vi "例7,1.vi"() -> ()   [LabVIEW 2017]
panel:
  out "7（X0=10.dx=2,Y）单条曲线":cluster{i32, i32, cluster{dbl[]}[]}(graph)
  out "6（X0=10.dx=2,Y）单条曲线":cluster{i32, i32, dbl[][]}(graph)
  out "5（X0=10.dx=2,Y）单条曲线":cluster{i32, i32, dbl[]}[](graph)
  out "4（X0=10.dx=2,Y）单条曲线":cluster{i32, i32, dbl[]}(graph)
  out "3（Y）单条曲线":cluster{dbl[]}[](graph)
  out "2（Y）多条曲线":dbl[][](graph)
  out "1（Y）单条曲线":dbl[](graph)
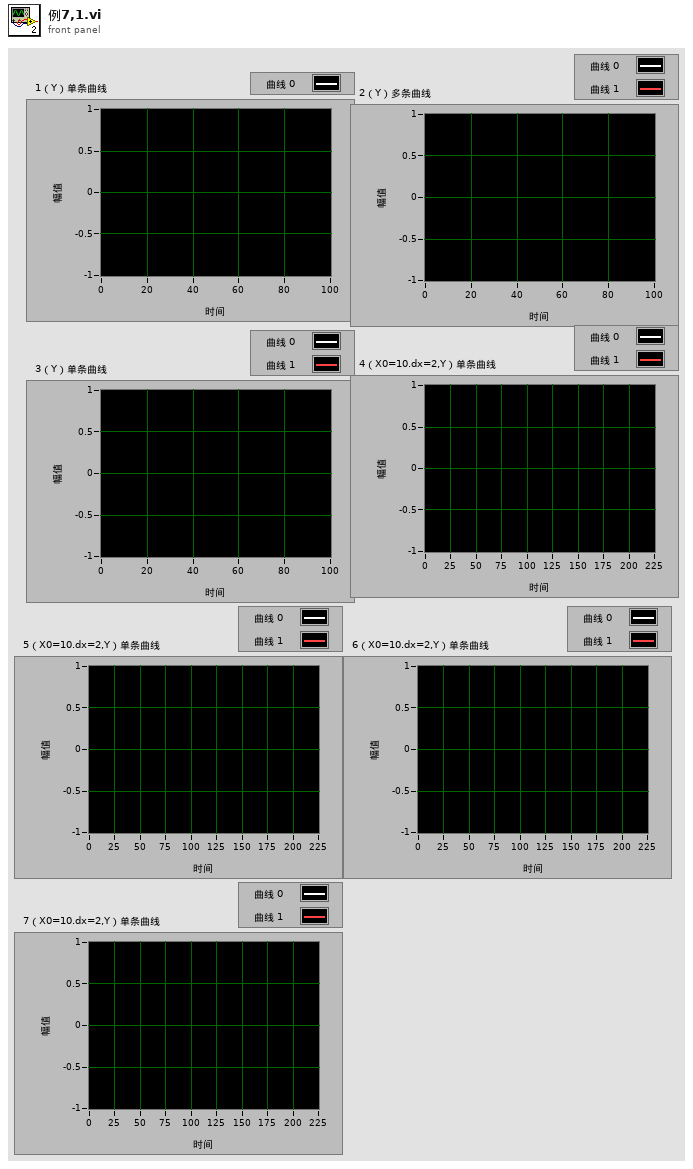
[diagram p1: front panel]
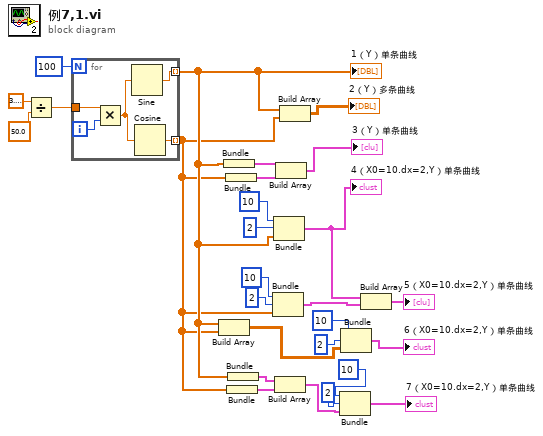
[diagram p0: block diagram]
diagram:
  n1 = Divide(x=3.141592653589793, y=50.0) -> (x/y=w25:dbl)
  n2 = for {
    N: 100 -> [_]
    tunnel: w25 -> [w31]
    tunnel: [w29] -> w19 mode=indexing
    tunnel: [w28] -> w23 mode=indexing
    i -> [w32]
    n3 = Multiply(x=w31, y=w32) -> (x*y=w30:dbl)
    n4 = Sine(x=w30) -> (sin(x)=w28:dbl)
    n5 = Cosine(x=w30) -> (cos(x)=w29:dbl)
  }
  "1（Y）单条曲线" <- w23
  n6 = Build Array(w23, w19) -> (w11:dbl[][])
  n7 = Bundle(w23) -> (w22:cluster{dbl[]})  [unwired: 1 in]
  n8 = Bundle(w19) -> (w21:cluster{dbl[]})  [unwired: 1 in]
  n9 = Bundle(w19) -> (w17:cluster{dbl[]})  [unwired: 1 in]
  n10 = Bundle(w23) -> (w18:cluster{dbl[]})  [unwired: 1 in]
  n11 = Bundle(10, 2, w19) -> (w8:cluster{i32, i32, dbl[]})  [unwired: 1 in]
  n12 = Bundle(10, 2, w23) -> (w12:cluster{i32, i32, dbl[]})  [unwired: 1 in]
  "4（X0=10.dx=2,Y）单条曲线" <- w12
  n13 = Build Array(w18, w17) -> (w16:cluster{dbl[]}[])
  n14 = Build Array(w22, w21) -> (→"3（Y）单条曲线":cluster{dbl[]}[])
  n15 = Build Array(w23, w19) -> (→"2（Y）多条曲线":dbl[][])
  n16 = Bundle(10, 2, w16) -> (→"7（X0=10.dx=2,Y）单条曲线":cluster{i32, i32, cluster{dbl[]}[]})  [unwired: 1 in]
  n17 = Bundle(10, 2, w11) -> (→"6（X0=10.dx=2,Y）单条曲线":cluster{i32, i32, dbl[][]})  [unwired: 1 in]
  n18 = Build Array(w12, w8) -> (→"5（X0=10.dx=2,Y）单条曲线":cluster{i32, i32, dbl[]}[])
